vi "QtoXML.vi"(1 "output cluster":T1, 2 "Actions":T2=[{"Toggle"=FALSE, "Open parameter editor"=FALSE, "Open MacroEditor"=FALSE, "Macro path"=path "", "Duration (s)"=0.0, "Parameters"=[{"Status"="", "Name"="", "Value"=0.0, "Changed"=FALSE}, {"Status"="", "Name"="", "Value"=0.0, "Changed"=FALSE}, {"Status"="", "Name"="", "Value"=0.0, "Changed"=FALSE}, {"Status"="", "Name"="", "Value"=0.0, "Changed"=FALSE}, {"Status"="", "Name"="", "Value"=0.0, "Changed"=FALSE}, {"Status"="", "Name"="", "Value"=0.0, "Changed"=FALSE}, {"Status"="", "Name"="", "Value"=0.0, "Changed"=FALSE}, {"Status"="", "Name"="", "Value"=0.0, "Changed"=FALSE}, {"Status"="", "Name"="", "Value"=0.0, "Changed"=FALSE}, {"Status"="", "Name"="", "Value"=0.0, "Changed"=FALSE}, {"Status"="", "Name"="", "Value"=0.0, "Changed"=FALSE}, {"Status"="", "Name"="", "Value"=0.0, "Changed"=FALSE}], "Comment"="", "Reps"=1}, {"Toggle"=FALSE, "Open parameter editor"=FALSE, "Open MacroEditor"=FALSE, "Macro path"=path "C:/Users/Student/Documents/LabVIEW Data/VIs/CuspControl/Sequences/Test2.mac", "Duration (s)"=0.0, "Parameters"=[{"Status"="", "Name"="", "Value"=0.0, "Changed"=FALSE}, {"Status"="", "Name"="", "Value"=0.0, "Changed"=FALSE}, {"Status"="", "Name"="", "Value"=0.0, "Changed"=FALSE}, {"Status"="", "Name"="", "Value"=0.0, "Changed"=FALSE}, {"Status"="", "Name"="", "Value"=0.0, "Changed"=FALSE}, {"Status"="", "Name"="", "Value"=0.0, "Changed"=FALSE}, {"Status"="", "Name"="", "Value"=0.0, "Changed"=FALSE}, {"Status"="", "Name"="", "Value"=0.0, "Changed"=FALSE}, {"Status"="", "Name"="", "Value"=0.0, "Changed"=FALSE}, {"Status"="", "Name"="", "Value"=0.0, "Changed"=FALSE}, {"Status"="", "Name"="", "Value"=0.0, "Changed"=FALSE}, {"Status"="", "Name"="", "Value"=0.0, "Changed"=FALSE}], "Comment"="", "Reps"=1}, {"Toggle"=TRUE, "Open parameter editor"=FALSE, "Open MacroEditor"=FALSE, "Macro path"=path "", "Duration (s)"=0.0, "Parameters"=[{"Status"="", "Name"="", "Value"=0.0, "Changed"=FALSE}, {"Status"="", "Name"="", "Value"=0.0, "Changed"=FALSE}, {"Status"="", "Name"="", "Value"=0.0, "Changed"=FALSE}, {"Status"="", "Name"="", "Value"=0.0, "Changed"=FALSE}, {"Status"="", "Name"="", "Value"=0.0, "Changed"=FALSE}, {"Status"="", "Name"="", "Value"=0.0, "Changed"=FALSE}, {"Status"="", "Name"="", "Value"=0.0, "Changed"=FALSE}, {"Status"="", "Name"="", "Value"=0.0, "Changed"=FALSE}, {"Status"="", "Name"="", "Value"=0.0, "Changed"=FALSE}, {"Status"="", "Name"="", "Value"=0.0, "Changed"=FALSE}, {"Status"="", "Name"="", "Value"=0.0, "Changed"=FALSE}, {"Status"="", "Name"="", "Value"=0.0, "Changed"=FALSE}], "Comment"="", "Reps"=1}] {"Reps" min=1 step=1; "Parameters"."Value" format="%_6p"; "Duration (s)" min=0.001 step=0.001 format="%_6p"}, 3 "XML File Path":path) -> ()   [LabVIEW 2018]
uses:
  Actions_arr.ctl
  Action.ctl
  Parameters.ctl
  <vilib>/Utility/xml.llb/Write to XML File(string).vi
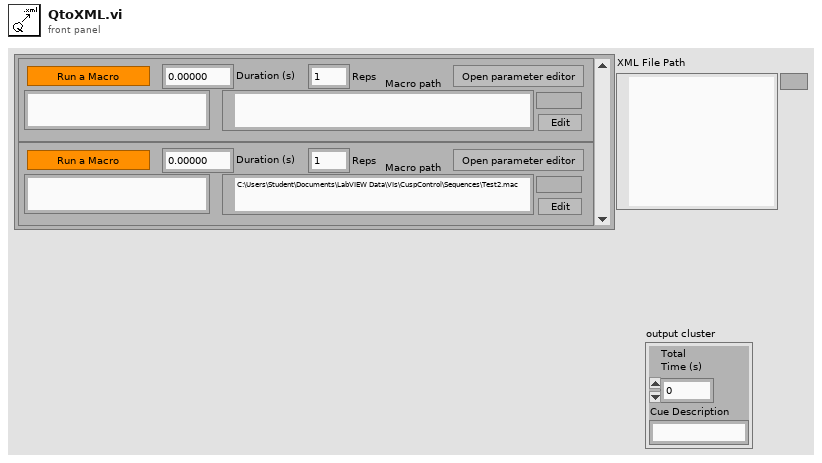
[diagram p1: front panel]
types:
  T1 = cluster{"Total\nTime (s)":dbl, "Cue Description":string}
  T2 = typedef "Actions_arr.ctl" = T3[]
  T3 = typedef "Action.ctl" = cluster{"Toggle":bool, "Open parameter editor":bool, "Open MacroEditor":bool, "Macro path":path, "Duration (s)":dbl, "Parameters":T4, "Comment":string, "Reps":i32}
  T4 = typedef "Parameters.ctl" = cluster{"Status":string, "Name":string, "Value":dbl, "Changed":bool}[]
  T5 = cluster{"Actions":T2, "output cluster":cluster{"Total\nTime (s)":dbl, "Cue Description":string}}
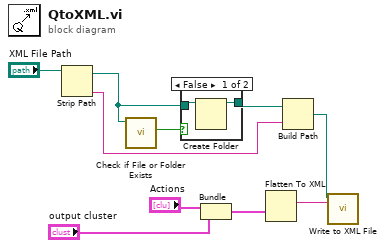
[diagram p0: block diagram]
diagram:
  n1 = Strip Path(path="XML File Path") -> (stripped path=w8:path, name=w6:string)
  n2 = call <vilib>:"Check if File or Folder Exists.vi"("path"=w8) -> ("file or folder exists?"=w9:bool)  [unwired: 8 in, 2 out]
  n3 = case shown="False" w9 {
    tunnel: w8 -> [w12 w13]
    tunnel: [w11 w13] -> w7
    frame False {
      n4 = Create Folder(path (use dialog)=w12) -> (created path=w11:path)  [unwired: 2 in, 2 out]
    }
    frame True {
    }
  }
  n5 = Bundle("Actions"="Actions", "output cluster"="output cluster") -> (w2:T5)  [unwired: 1 in]
  n6 = Flatten To XML(anything=w2) -> (xml string=w10:string)
  n7 = Build Path(base path=w7, name or relative path=w6) -> (appended path=w5:path)
  n8 = call-poly <vilib>:"Write to XML File.vi"("XML Input"=w10, "XML File Path"=w5) -> ()  [unwired: 7 in, 3 out]
